vi "SetValueType.vi"(0 "variant":variant, 5 "valuetype":T1, 11 "error in":errorcluster) -> (4 "variant out":variant, 15 "error out":errorcluster)   [LabVIEW 2019]
uses:
  Valuetype.ctl
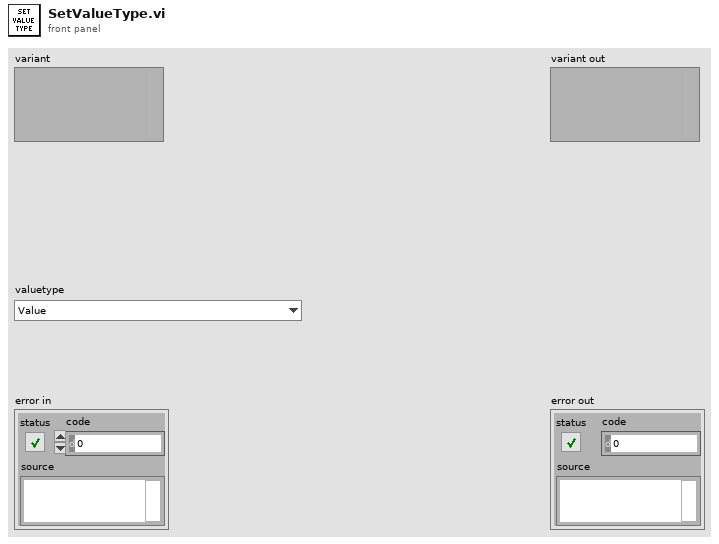
[diagram p1: front panel]
types:
  T1 = typedef "Valuetype.ctl" = enum16{"Value", "Variable", "Function"}
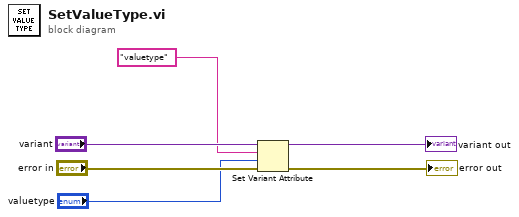
[diagram p0: block diagram]
diagram:
  n1 = Set Variant Attribute(Variant="variant", name="valuetype", value="valuetype", error in="error in") -> (Variant out=→"variant out":variant, error out=→"error out":errorcluster)  [unwired: 1 out]
